vi "Экзамен камень-ножницы-бумага доп.vi"() -> ()   [LabVIEW 2021]
panel:
  out "Вы":string
  out "String":string
  out "Компьютер":string
  out "Состояние":T1
  in  "Камень":bool
  in  "Бумага":bool
  in  "Ножницы":bool
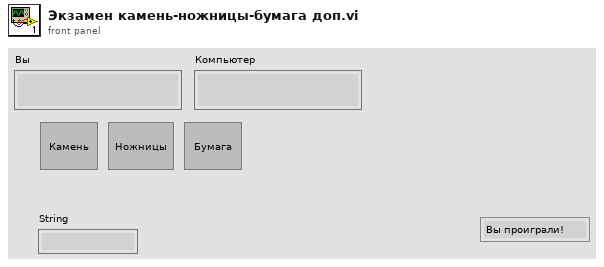
[diagram p1: front panel]
types:
  T1 = typedef "Экз1.ctl" = enum16{"Вы проиграли!", "Ничья!", "Вы победили!", "БумагаП-БумагаК", "НожницыП-БумагаК", "КаменьП-БумагаК", "БумагаП-НожницыК", "НожницыП-НожницыК", "КаменьП-НожницыК", "БумагаП-КаменьК", "НожницыП-КаменьК", "КаменьП-КаменьК", "Играем!"}
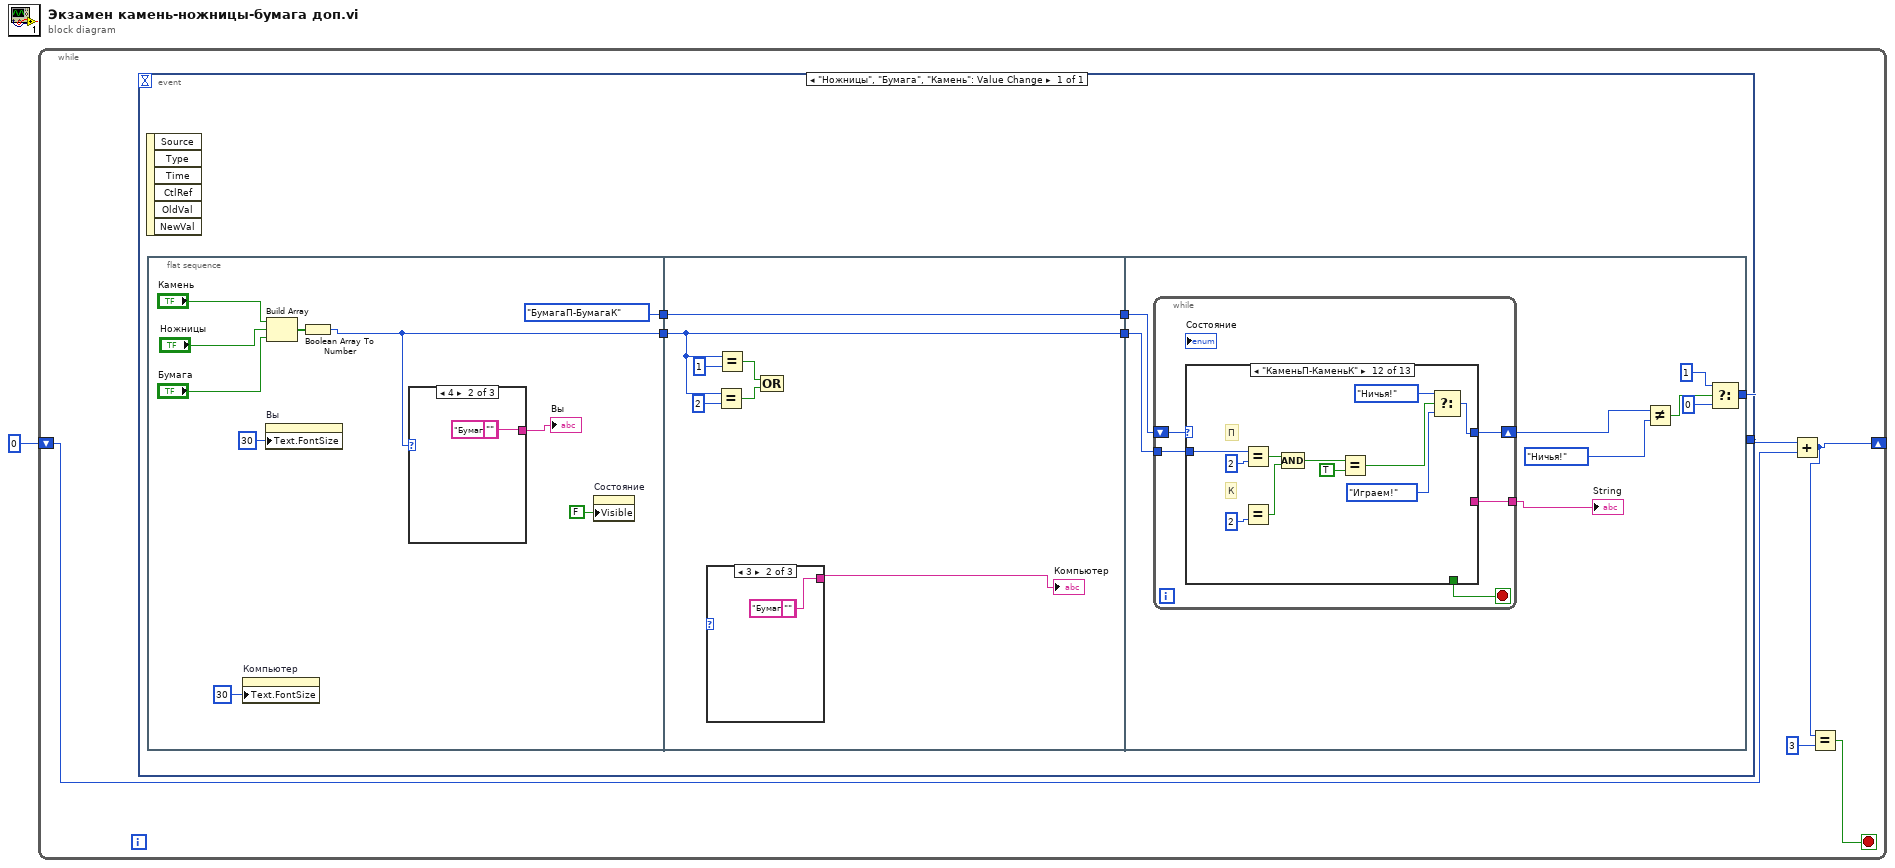
[diagram p0: block diagram]
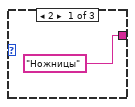
[diagram p2: hidden frame]
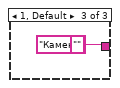
[diagram p3: hidden frame]
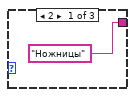
[diagram p4: hidden frame]
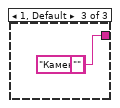
[diagram p5: hidden frame]
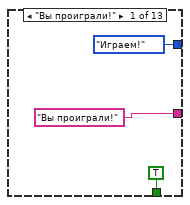
[diagram p6: hidden frame]
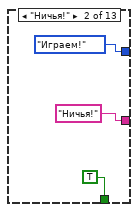
[diagram p7: hidden frame]
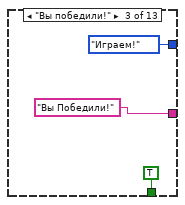
[diagram p8: hidden frame]
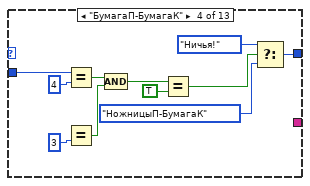
[diagram p9: hidden frame]
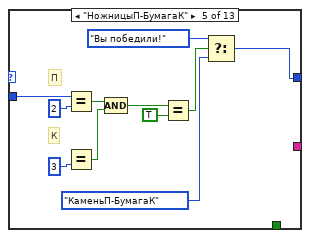
[diagram p10: hidden frame]
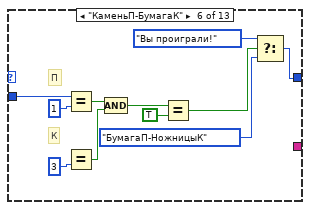
[diagram p11: hidden frame]
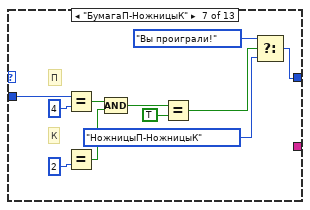
[diagram p12: hidden frame]
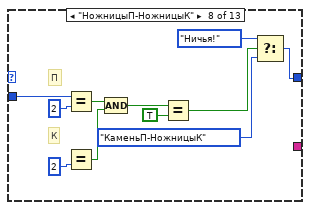
[diagram p13: hidden frame]
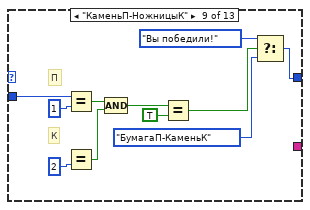
[diagram p14: hidden frame]
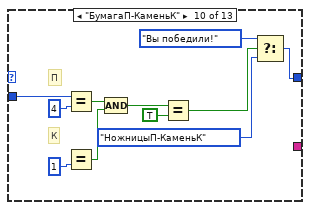
[diagram p15: hidden frame]
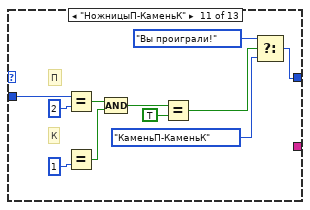
[diagram p16: hidden frame]
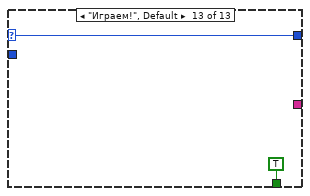
[diagram p17: hidden frame]
diagram:
  n1 = while {
    shift-right: [w4] -> _
    shift-left: 0 -> [w5]
    stop <- w2 stop-if-true
    n2 = event shown="[0] \"Ножницы\", \"Бумага\", \"Камень\": Value Change" {
      selector: _ -> [_]
      dyn-events: _ -> [_]
      timeout: _ -> [_]
      tunnel: [w11] -> w6
      event "Ножницы", "Бумага", "Камень": Value Change {
        n3 = event-data() -> ()  [unwired: 1 in, 6 out]
        n4 = flat-sequence {
          tunnel: [w15] -> w10
          tunnel: [Экз1."БумагаП-БумагаК" ("Состояние")] -> w8
          tunnel: w10 -> [w28]
          tunnel: [w28] -> w9
          tunnel: w8 -> [w31]
          tunnel: [w31] -> w7
          tunnel: w9 -> [w43]
          tunnel: w7 -> [w42]
          tunnel: [w35] -> w11
          frame #0 {
            n5 = property on="Компьютер" class="Str"("Text.FontSize"=u32 30 ("Text.Font:Size")) -> ()  [unwired: 2 in, 2 out]
            n6 = property on="Вы" class="Str"("Text.FontSize"=u32 30 ("Text.Font:Size")) -> ()  [unwired: 2 in, 2 out]
            n7 = Build Array("Камень", "Ножницы", "Бумага") -> (w21:bool[])
            n8 = Boolean Array To Number(Boolean array=w21) -> (number=w15:u32)
            n9 = case shown="4" w15 {
              tunnel: ["Ножницы" ("Компьютер") "Бумага" ("Компьютер") "Камень" ("Компьютер")] -> w14
              frame 2 {
              }
              frame 4 {
                (unwired) "" ("Компьютер")
              }
              frame 1, Default {
                (unwired) "" ("Компьютер")
              }
            }
            "Вы" <- w14
            n10 = property on="Состояние" class="Enum (strict)"("Visible"=FALSE) -> ()  [unwired: 2 in, 2 out]
          }
          frame #1 {
            n11 = case shown="3" {
              selector: _ -> [_ _ _]
              tunnel: ["Ножницы" ("Компьютер") "Бумага" ("Компьютер") "Камень" ("Компьютер")] -> w30
              frame 2 {
              }
              frame 3 {
                (unwired) "" ("Компьютер")
              }
              frame 1, Default {
                (unwired) "" ("Компьютер")
              }
            }
            "Компьютер" <- w30
            n12 = Equal?(x=w28, y=u32 2) -> (x = y?=w25:bool)
            n13 = Equal?(x=w28, y=u32 1) -> (x = y?=w26:bool)
            n14 = Compound Arithmetic op=OR(w26, w25) -> ()  [unwired: 1 out]
          }
          frame #2 {
            n15 = while {
              tunnel: w43 -> [w47]
              shift-right: [w48] -> w40
              shift-left: w42 -> [w46]
              tunnel: [w44] -> w41
              stop <- w45 stop-if-true
              n16 = case shown="\"КаменьП-КаменьК\"" w46 {
                selector: w46 -> [_ _ _ _ _ _ _ _ _ _ _ _ w158]
                tunnel: w47 -> [_ _ _ w68 w79 w90 w101 w112 w123 w134 w145 w156 _]
                tunnel: [Экз1."Играем!" ("Состояние") Экз1."Играем!" ("Состояние") Экз1."Играем!" ("Состояние") w58 w72 w83 w94 w105 w116 w127 w138 w149 w158] -> w48
                tunnel: [TRUE TRUE TRUE _ _ _ _ _ _ _ _ _ TRUE] -> w45
                tunnel: ["Вы проиграли!" ("String") "Ничья!" ("String") "Вы Победили!" ("String") _ _ _ _ _ _ _ _ _ _] -> w44
                frame "Вы проиграли!" {
                }
                frame "Ничья!" {
                }
                frame "Вы победили!" {
                }
                frame "БумагаП-БумагаК" {
                  n17 = Equal?(x=w68, y=u32 4) -> (x = y?=w65:bool)
                  n18 = Equal?(y=u32 3) -> (x = y?=w64:bool)  [unwired: 1 in]
                  n19 = Compound Arithmetic op=AND(w65, w64) -> (w63:bool)
                  n20 = Equal?(x=w63, y=TRUE) -> (x = y?=w61:bool)
                  n21 = Select(t=Экз1."Ничья!" ("Состояние"), s=w61, f=Экз1."НожницыП-БумагаК" ("Состояние")) -> (s? t:f=w58:T1)
                }
                frame "НожницыП-БумагаК" {
                  # "К"
                  # "П"
                  n22 = Equal?(x=w79, y=u32 2) -> (x = y?=w74:bool)
                  n23 = Equal?(y=u32 3) -> (x = y?=w73:bool)  [unwired: 1 in]
                  n24 = Compound Arithmetic op=AND(w74, w73) -> (w76:bool)
                  n25 = Equal?(x=w76, y=TRUE) -> (x = y?=w69:bool)
                  n26 = Select(t=Экз1."Вы победили!" ("Состояние"), s=w69, f=Экз1."КаменьП-БумагаК" ("Состояние")) -> (s? t:f=w72:T1)
                }
                frame "КаменьП-БумагаК" {
                  # "К"
                  # "П"
                  n27 = Equal?(x=w90, y=u32 1) -> (x = y?=w85:bool)
                  n28 = Equal?(y=u32 3) -> (x = y?=w84:bool)  [unwired: 1 in]
                  n29 = Compound Arithmetic op=AND(w85, w84) -> (w87:bool)
                  n30 = Equal?(x=w87, y=TRUE) -> (x = y?=w80:bool)
                  n31 = Select(t=Экз1."Вы проиграли!" ("Состояние"), s=w80, f=Экз1."БумагаП-НожницыК" ("Состояние")) -> (s? t:f=w83:T1)
                }
                frame "БумагаП-НожницыК" {
                  # "К"
                  # "П"
                  n32 = Equal?(x=w101, y=u32 4) -> (x = y?=w96:bool)
                  n33 = Equal?(y=u32 2) -> (x = y?=w95:bool)  [unwired: 1 in]
                  n34 = Compound Arithmetic op=AND(w96, w95) -> (w98:bool)
                  n35 = Equal?(x=w98, y=TRUE) -> (x = y?=w91:bool)
                  n36 = Select(t=Экз1."Вы проиграли!" ("Состояние"), s=w91, f=Экз1."НожницыП-НожницыК" ("Состояние")) -> (s? t:f=w94:T1)
                }
                frame "НожницыП-НожницыК" {
                  # "К"
                  # "П"
                  n37 = Equal?(x=w112, y=u32 2) -> (x = y?=w107:bool)
                  n38 = Equal?(y=u32 2) -> (x = y?=w106:bool)  [unwired: 1 in]
                  n39 = Compound Arithmetic op=AND(w107, w106) -> (w109:bool)
                  n40 = Equal?(x=w109, y=TRUE) -> (x = y?=w102:bool)
                  n41 = Select(t=Экз1."Ничья!" ("Состояние"), s=w102, f=Экз1."КаменьП-НожницыК" ("Состояние")) -> (s? t:f=w105:T1)
                }
                frame "КаменьП-НожницыК" {
                  # "К"
                  # "П"
                  n42 = Equal?(x=w123, y=u32 1) -> (x = y?=w118:bool)
                  n43 = Equal?(y=u32 2) -> (x = y?=w117:bool)  [unwired: 1 in]
                  n44 = Compound Arithmetic op=AND(w118, w117) -> (w120:bool)
                  n45 = Equal?(x=w120, y=TRUE) -> (x = y?=w113:bool)
                  n46 = Select(t=Экз1."Вы победили!" ("Состояние"), s=w113, f=Экз1."БумагаП-КаменьК" ("Состояние")) -> (s? t:f=w116:T1)
                }
                frame "БумагаП-КаменьК" {
                  # "К"
                  # "П"
                  n47 = Equal?(x=w134, y=u32 4) -> (x = y?=w129:bool)
                  n48 = Equal?(y=u32 1) -> (x = y?=w128:bool)  [unwired: 1 in]
                  n49 = Compound Arithmetic op=AND(w129, w128) -> (w131:bool)
                  n50 = Equal?(x=w131, y=TRUE) -> (x = y?=w124:bool)
                  n51 = Select(t=Экз1."Вы победили!" ("Состояние"), s=w124, f=Экз1."НожницыП-КаменьК" ("Состояние")) -> (s? t:f=w127:T1)
                }
                frame "НожницыП-КаменьК" {
                  # "К"
                  # "П"
                  n52 = Equal?(x=w145, y=u32 2) -> (x = y?=w140:bool)
                  n53 = Equal?(y=u32 1) -> (x = y?=w139:bool)  [unwired: 1 in]
                  n54 = Compound Arithmetic op=AND(w140, w139) -> (w142:bool)
                  n55 = Equal?(x=w142, y=TRUE) -> (x = y?=w135:bool)
                  n56 = Select(t=Экз1."Вы проиграли!" ("Состояние"), s=w135, f=Экз1."КаменьП-КаменьК" ("Состояние")) -> (s? t:f=w138:T1)
                }
                frame "КаменьП-КаменьК" {
                  # "К"
                  # "П"
                  n57 = Equal?(x=w156, y=u32 2) -> (x = y?=w151:bool)
                  n58 = Equal?(y=u32 2) -> (x = y?=w150:bool)  [unwired: 1 in]
                  n59 = Compound Arithmetic op=AND(w151, w150) -> (w153:bool)
                  n60 = Equal?(x=w153, y=TRUE) -> (x = y?=w146:bool)
                  n61 = Select(t=Экз1."Ничья!" ("Состояние"), s=w146, f=Экз1."Играем!" ("Состояние")) -> (s? t:f=w149:T1)
                }
                frame "Играем!", Default {
                }
              }
            }
            "String" <- w41
            n62 = Not Equal?(x=w40, y=Экз1."Ничья!" ("Состояние")) -> (x != y?=w38:bool)
            n63 = Select(t=1, s=w38, f=0) -> (s? t:f=w35:i32)
          }
        }
      }
    }
    n64 = Add(x=w6, y=w5) -> (x+y=w4:i32)
    n65 = Equal?(x=w4, y=3) -> (x = y?=w2:bool)
  }
